vi "Log Error.vi"(8 "error in (no error)":errorcluster, 10 "Error Data":T1, 11 "Elevator Controller in":refnum<class "Elevator Controller.lvclass">) -> (0 "error out":errorcluster, 3 "Elevator Controller out":refnum<class "Elevator Controller.lvclass">)   [LabVIEW 2019, in "Elevator Controller.lvlib" / "Elevator Controller.lvclass"]
uses:
  Elevator Controller.lvclass
  Error Level -enum.ctl
  Error Data.ctl
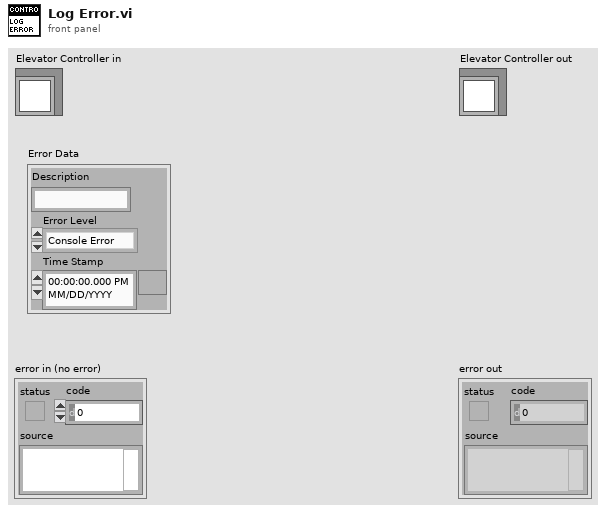
[diagram p1: front panel]
types:
  T1 = typedef "Elevator Controller.lvlib/Elevator Controller.lvclass/Error Data.ctl" = cluster{"Description":string, "Error Level":T2, "Time Stamp":timestamp}
  T2 = typedef "Elevator Controller.lvlib/Elevator Controller.lvclass/Error Level -enum.ctl" = enum16{"Console Error", "Sensor Interface IO Error", "Process Step Error"}
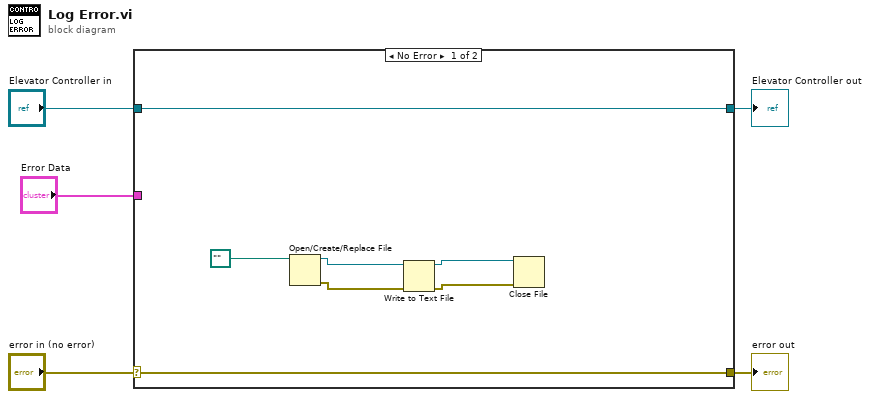
[diagram p0: block diagram]
diagram:
  n1 = case shown="No Error" "error in (no error)" {
    selector: "error in (no error)" -> [w11 w14]
    tunnel: [w11 w14] -> w4
    tunnel: [w12 w13] -> w2
    tunnel: "Elevator Controller in" -> [w12 w13]
    tunnel: "Error Data" -> [_ _]
    frame No Error {
      n2 = Open/Create/Replace File(file path (use dialog)=path "") -> (refnum out=w8:refnum<file>, error out=w10:errorcluster)  [unwired: 5 in, 1 out]
      n3 = Write to Text File(file (use dialog)=w8, error in=w10) -> (refnum out=w7:refnum<file>, error out=w9:errorcluster)  [unwired: 2 in, 1 out]
      n4 = Close File(refnum=w7, error in=w9) -> ()  [unwired: 2 out]
    }
    frame Error {
    }
  }
  "error out" <- w4
  "Elevator Controller out" <- w2
